vi "enable control.vi"(6 "Enable ?":bool, 8 "error in":errorcluster, 11 "Control":refnum<vi>[](array[refnum])) -> (0 "error out":errorcluster)   [LabVIEW 2017]
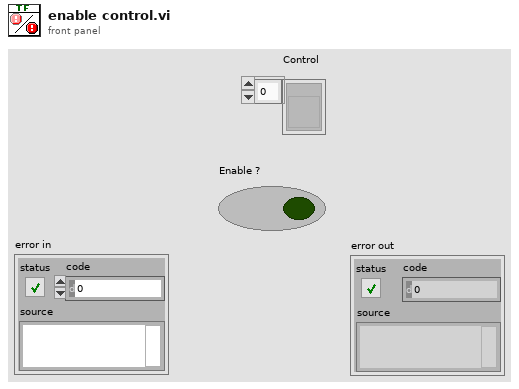
[diagram p1: front panel]
types:
  T1 = enum8{"Enabled", "Disabled", "Disabled and Grayed Out"}
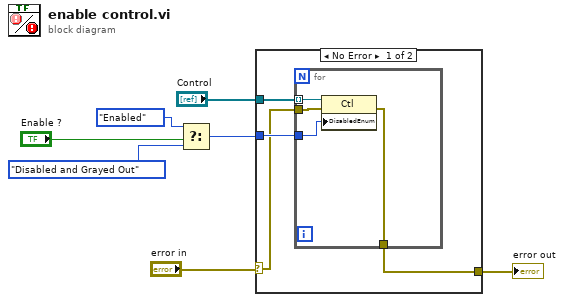
[diagram p0: block diagram]
diagram:
  n1 = Select(t=T1."Enabled" ("Disabled"), s="Enable ?", f=T1."Disabled and Grayed Out" ("Disabled")) -> (s? t:f=w4:T1)
  n2 = case shown="No Error" "error in" {
    selector: "error in" -> [w9 w16]
    tunnel: "Control" -> [w11 _]
    tunnel: w4 -> [w10 _]
    tunnel: [w8 w16] -> w1
    frame No Error {
      n3 = for {
        tunnel: w11 -> [w15] mode=indexing
        tunnel: w10 -> [w14]
        tunnel: w9 -> [w13]
        tunnel: [w12] -> w8
        n4 = property class="Ctl"(reference=w15, error in=w13, "DisabledEnum"=w14) -> (error out=w12:errorcluster)  [unwired: 1 out]
      }
    }
    frame Error {
    }
  }
  "error out" <- w1
